vi "Notifier-with-memory-string.vi"(8 "error in":errorcluster, 10 "Timeout [ms]":i32, 11 "Notifier in":refnum<notifier>) -> (0 "error IO":errorcluster, 2 "Notification":string)   [LabVIEW 2013, in "CameraVision.lvlib" / "CV-UI.lvclass"]
uses:
  CV-UI.lvclass
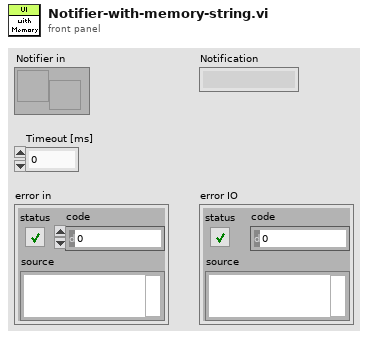
[diagram p1: front panel]
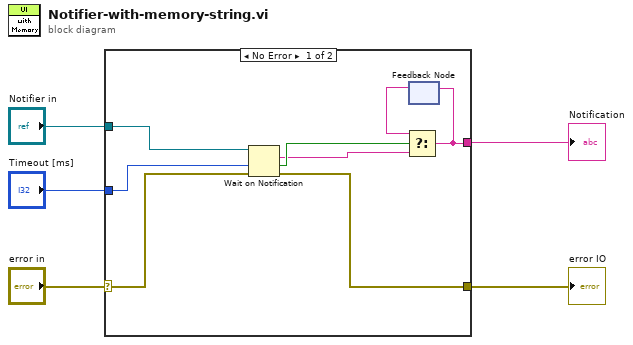
[diagram p0: block diagram]
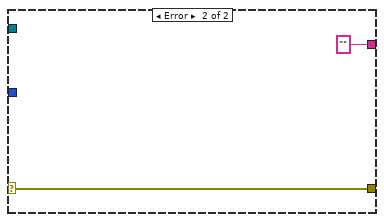
[diagram p2: hidden frame]
diagram:
  n1 = case shown="No Error" "error in" {
    selector: "error in" -> [w6 w15]
    tunnel: [w13 w15] -> w5
    tunnel: "Timeout [ms]" -> [w12 _]
    tunnel: "Notifier in" -> [w11 _]
    tunnel: [w7 ""] -> w2
    frame No Error {
      n2 = Wait on Notification(notifier=w11, timeout in ms (-1)=w12, error in (no error)=w6) -> (notification=w9:string, timed out?=w10:bool, error out=w13:errorcluster)  [unwired: 1 in, 1 out]
      n3 = feedback #1() -> (w8:string)  [unwired: 1 in]
      n4 = Select(t=w8, s=w10, f=w9) -> (s? t:f=w7:string)
      n5 = feedback-in #1(w7) -> ()
    }
    frame Error {
    }
  }
  "Notification" <- w2
  "error IO" <- w5
